vi "DataBase - Top VI.vi"(8 "error in":errorcluster) -> (0 "error out":errorcluster)   [LabVIEW 2024, in "Data Base.lvlib"]
uses:
  Data Base.lvlib
  DataBase Queue - Dequeue.vi
  User Interface/UI Queue - Enqueue.vi
  DataBase Queue - Enqueue.vi
  DataBase Queue - Destroy.vi
  User Interface/User Interface.lvlib
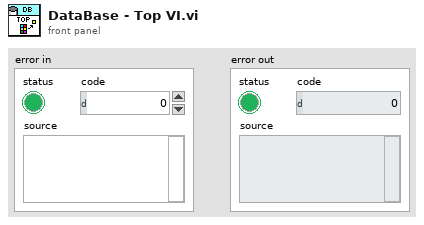
[diagram p1: front panel]
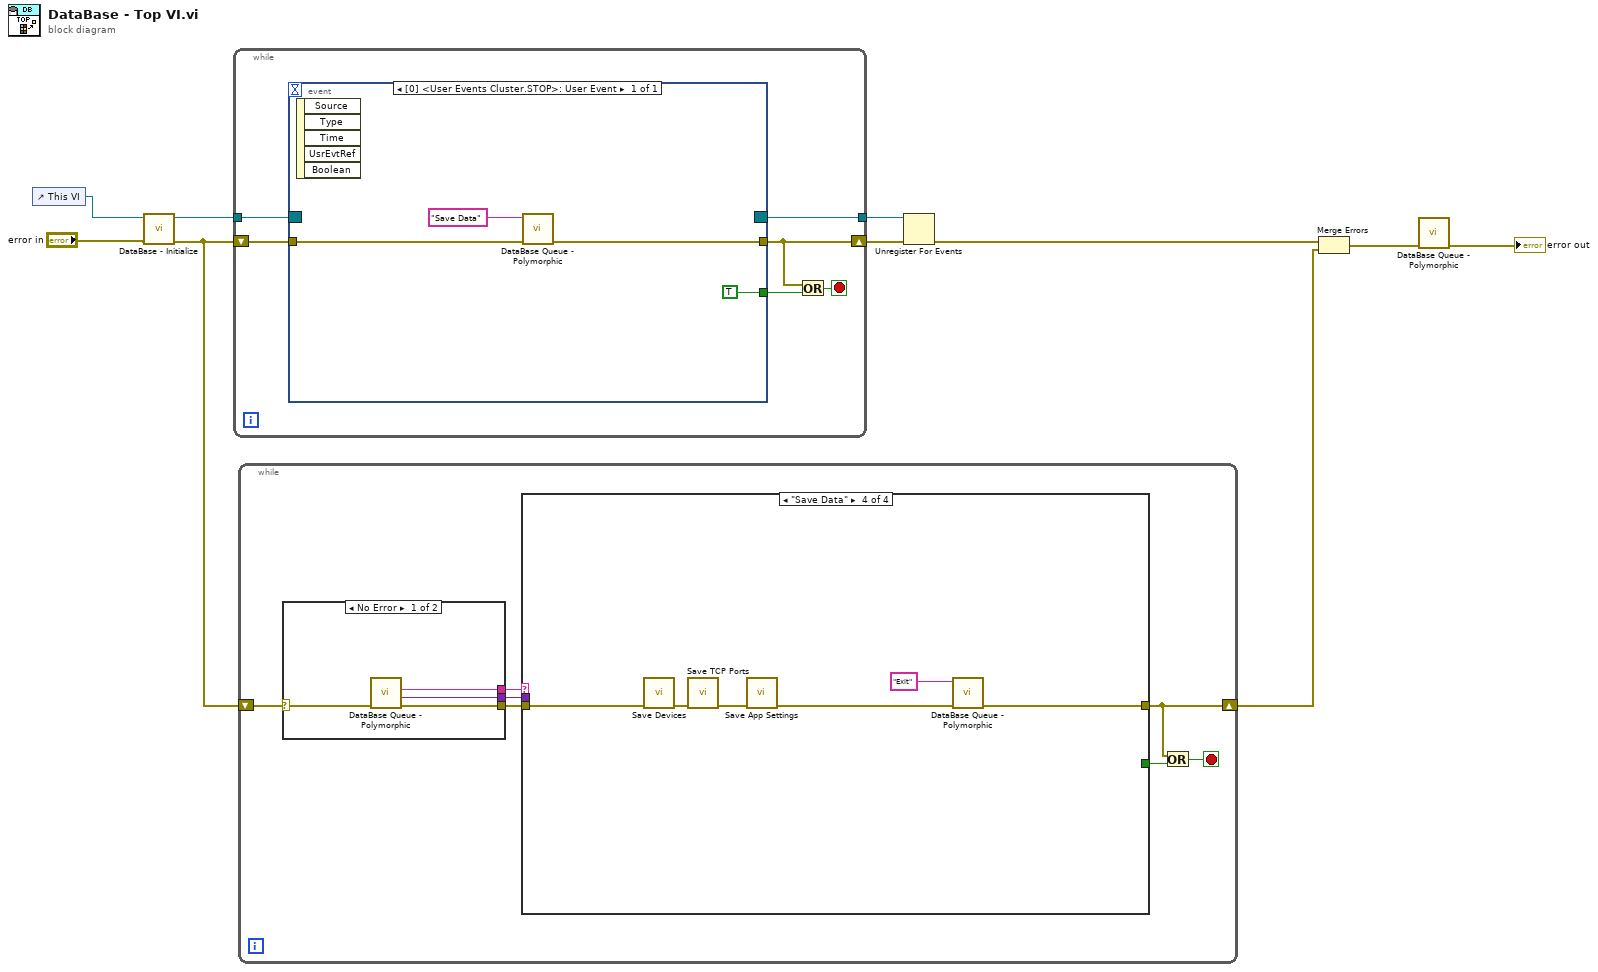
[diagram p0: block diagram]
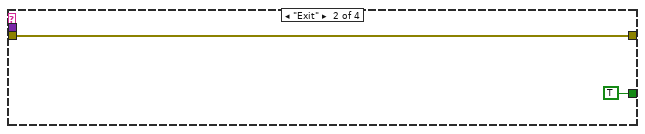
[diagram p3: hidden frame]
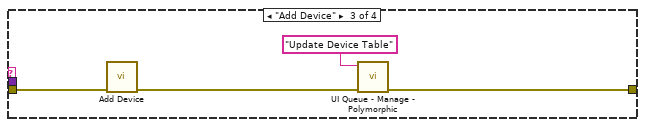
[diagram p4: hidden frame]
diagram:
  n1 = control-ref of="This VI"() -> (w10:refnum<vi>)
  n2 = call "DataBase - Initialize.vi"("error in (no error)"="error in", "VI In"=w10) -> ("error out"=w5:errorcluster, "Event Registration Out"=w8:refnum<event-registration>)  [unwired: 8 in]
  n3 = while {
    tunnel: w8 -> [w16]
    shift-right: [w11] -> w7
    shift-left: w5 -> [w15]
    tunnel: [w14] -> w6
    stop <- w12 stop-if-true
    n4 = event shown="[0] <User Events Cluster.STOP>: User Event" {
      selector: w16 -> [_]
      dyn-events: [_] -> w14
      timeout: _ -> [_]
      tunnel: w15 -> [w20]
      tunnel: [w19] -> w11
      tunnel: [TRUE] -> w13
      event User Event {
        n5 = event-data() -> ()  [unwired: 1 in, 5 out]
        n6 = call-poly "DataBase Queue - Polymorphic.vi"("error in"=w20, "Message"="Save Data") -> ("error out"=w19:errorcluster)  [unwired: 9 in]
      }
    }
    n7 = Or(x=w11, y=w13) -> (x .or. y?=w12:bool)
  }
  n8 = while {
    shift-right: [w21] -> w3
    shift-left: w5 -> [w27]
    stop <- w22 stop-if-true
    n9 = case shown="No Error" w27 {
      selector: w27 -> [w41 w45]
      tunnel: [w42 w45] -> w24
      tunnel: [w44 _] -> w26
      tunnel: [w43 _] -> w25
      frame No Error {
        n10 = call-poly "DataBase Queue - Polymorphic.vi"("error in"=w41) -> ("error out"=w42:errorcluster, "Message Data"=w43:variant, "Message"=w44:string)  [unwired: 8 in]
      }
      frame Error {
      }
    }
    n11 = case shown="\"Save Data\"" w26 {
      tunnel: w25 -> [_ _ _ _]
      tunnel: w24 -> [w28 w29 w34 w38]
      tunnel: [w28 w29 w31 w39] -> w21
      tunnel: [_ TRUE _ _] -> w23
      frame "IDLE", Default {
      }
      frame "Exit" {
      }
      frame "Add Device" {
        n12 = call "Add Device.vi"("error in"=w34) -> ("error out"=w32:errorcluster)  [unwired: 10 in]
        n13 = call-poly "UI Queue - Manage - Polymorphic.vi"("error in"=w32, "Message"="Update Device Table") -> ("error out"=w31:errorcluster)  [unwired: 9 in]
      }
      frame "Save Data" {
        n14 = call "Save Devices.vi"("error in"=w38) -> ("error out"=w37:errorcluster)  [unwired: 10 in]
        n15 = call "Save TCP Ports.vi"("error in"=w37) -> ("error out"=w36:errorcluster)  [unwired: 10 in]
        n16 = call "Save App Settings.vi"("error in (no error)"=w36) -> ("error out"=w35:errorcluster)  [unwired: 10 in]
        n17 = call-poly "DataBase Queue - Polymorphic.vi"("error in"=w35, "Message"="Exit") -> ("error out"=w39:errorcluster)  [unwired: 9 in]
      }
    }
    n18 = Or(x=w21, y=w23) -> (x .or. y?=w22:bool)
  }
  n19 = Unregister For Events(event registration refnum=w6, error in=w7) -> (error out=w4:errorcluster)
  n20 = Merge Errors(w4, w3) -> (w2:errorcluster)
  n21 = call-poly "DataBase Queue - Polymorphic.vi"("error in"=w2) -> ("error out"=→"error out":errorcluster)  [unwired: 10 in]
